vi "status of robot.vi"() -> ()   [LabVIEW 2020]
panel:
  out "status of robot":bool
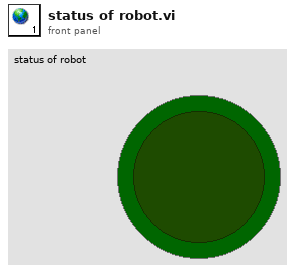
[diagram p1: front panel]
diagram:
